vi "Main.vi"   [LabVIEW 2020]
doc: "Main interface to Dataflow DJ.\n\n<b>Execution System:</b> User Interface"
uses:
  Libraries/User Interface/Sub Panels Cluster.ctl
  Libraries/Track Info/Track Info FGV Enum.ctl
  Libraries/Audio Output/Audio Output Queue Type.ctl
  Libraries/Config File/Config Cluster.ctl
  Libraries/Track Info/Track Info.ctl
  <vilib>/Analysis/1siggen.llb/Ramp Pattern by Samples.vi
  Packed Libraries/Globals.lvlibp/Constants.vi
  <vilib>/Platform/TimedLoop/scheduler/LVUserAPI/_suppVIs/Create_SoftwareTrigger_TSource.vi
  Libraries/Audio Engine/Audio Engine.lvlib
  Libraries/Audio Output/Audio Output.lvlib
  Packed Libraries/Globals.lvlibp
  Libraries/User Interface/User Interface.lvlib
  Libraries/Config File/Config File.lvlib
  Libraries/Track Info/Track Info.lvlib
  <vilib>/Analysis/NI_AALBase.lvlib
  Plugin Interfaces/Controller Interface/Controller Interface.lvlibp/Controller Interface Class/Controller Interface.lvclass
  Libraries/Audio Recording/Audio Recording.lvlib
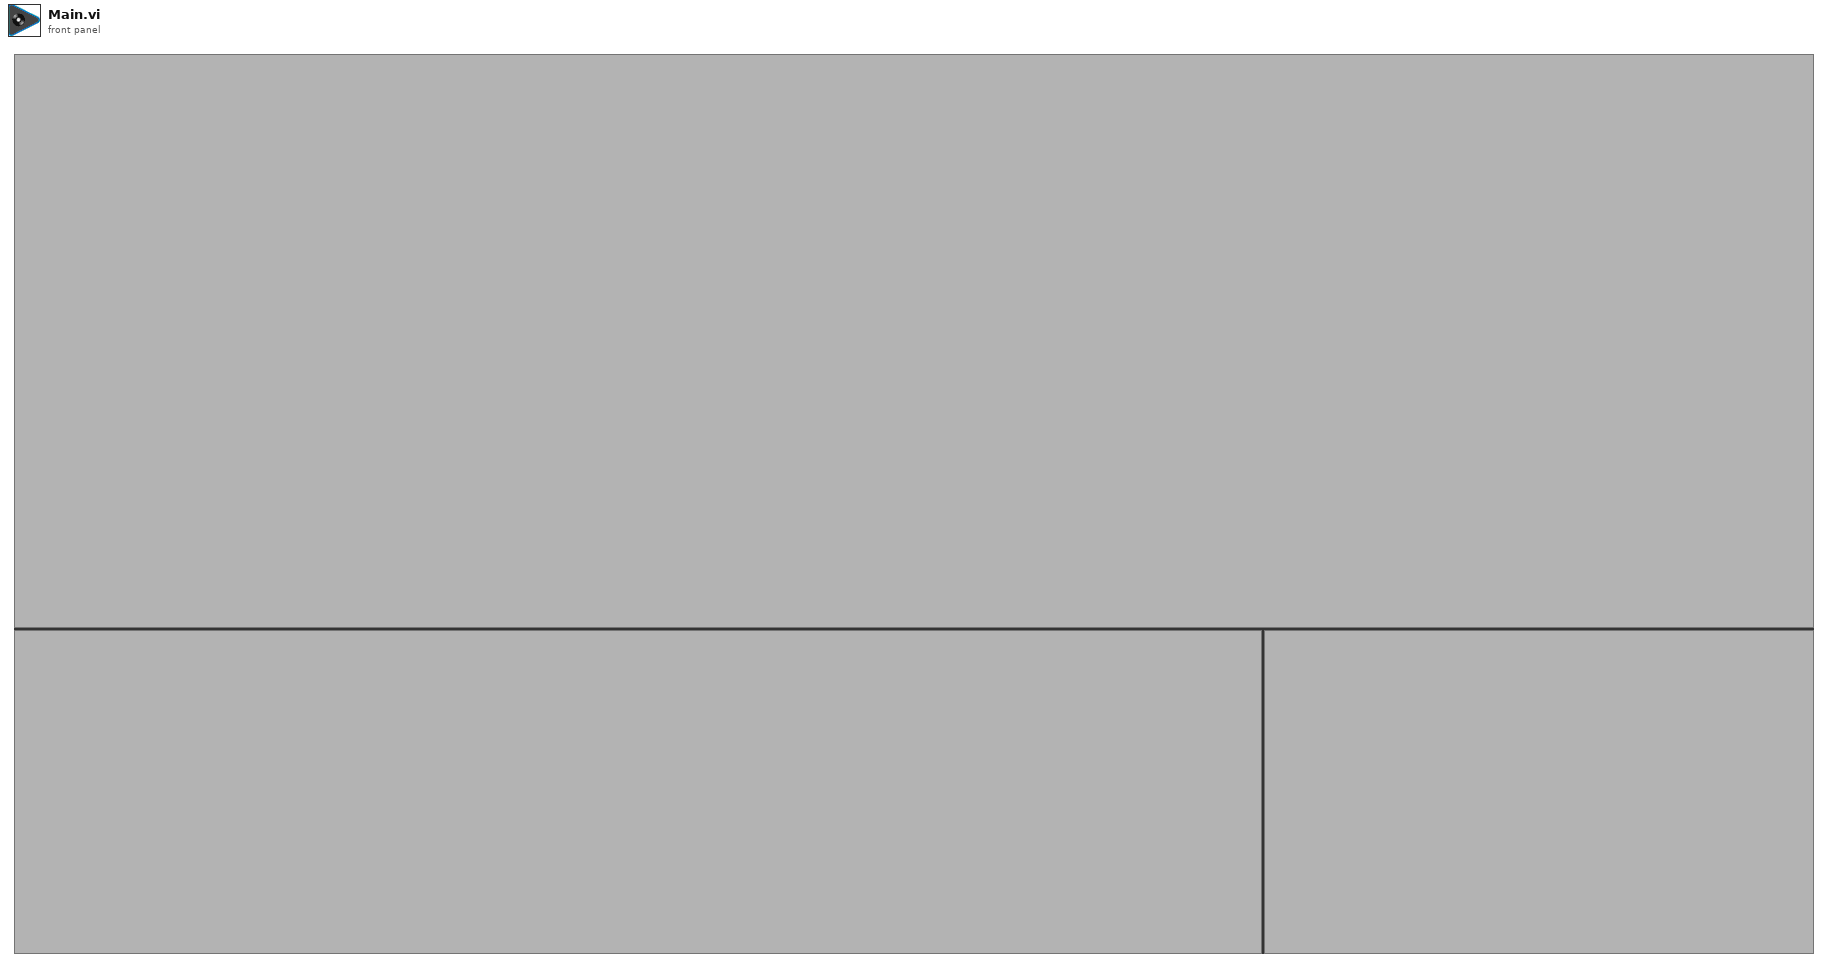
[diagram p1: front panel]
types:
  T1 = typedef "User Interface.lvlib/Sub Panels Cluster.ctl" = cluster{"DJ Interface":refnum<vi>, "File Browser":refnum<vi>, "Audio Config":refnum<vi>}
  T2 = typedef "Track Info.lvlib/Track Info FGV Enum.ctl" = enum16{"Init", "Update Track", "Update Multiple Tracks", "Get Track", "Get Multiple Tracks"}
  T3 = typedef "Config File.lvlib/Config Cluster.ctl" = cluster{"Track Info":T4[]}
  T4 = typedef "Track Info.lvlib/Track Info.ctl" = cluster{"Path":path, "Length (Samples)":i32, "Channels":i32, "Sample Rate (Hz)":i32, "BPM":dbl, "Cue Points (Samples)":i32[]}
  T5 = typedef "Audio Output.lvlib/Audio Output Queue Type.ctl" = cluster{"Master":waveform(i16)[], "Headphones":waveform(i16)[], "Start Time":dbl, "Record":bool}
  T6 = enum32{"invalid app kind", "Development System", "Run Time System", "Student Edition", "Embedded LabVIEW", "Evaluation", "Custom"}
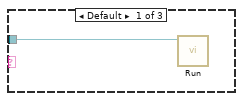
[diagram p2: hidden frame]
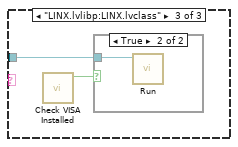
[diagram p4: hidden frame]
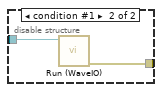
[diagram p7: hidden frame]
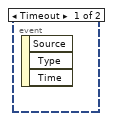
[diagram p8: hidden frame]
diagram:
  w12 = FALSE  # Shutdown
  # "#TODO\nOffload this checking logic to the class itself"
  # "Load WaveIO VIs programmatically\n\nif waveio.dll exists, then dynamically call VIs in waveio.llb\nif it doesn't exist, fall back to lvsound2.dll\n\nshould also address this issue"
  # "Startup order required\nAudio Processing\n- Setup message queues for all control messages from UI and hardware\n- Begin generating output data\nAutio Output\n- Setup message queue from audio config UI panel\nUser Interface (DJ Interface)\n- Setup message queue to receive UI changes\n- Scan all UI elements and send values and limits to Audio Processing\nHardware Controller\n- Setup hardware and read current IO state\n- Send IO state to Audio Processing, which will then relay changes back to UI\n\n#TODO Use named Notifiers to wait for each component to start up"
  # "EXECUTION SYSTEMS\n\nAudio Processing.Run.vi    Standard\nAudio Output.Run.vi    Instrument I/O\nMain.vi    User Interface\nUser Interface.DJ Interface.vi    User Interface\nUser Interface.File Browser.vi    User Interface\nUser Interface.Audio Config.vi    User Interface\nHardware Control.DAQmx Run.vi    Data Acquisition\nAudio File Input.Load Async.vi    Other 1"
  # "Dataflow DJ Mixer- A multichannel audio mixing application written entirely in LabVIEW, based on Dataflow DJ.\n    Copyright (C) 2020  Dataflow G\n    \n    This program is free software: you can redistribute it and/or modify\n    it under the terms of the GNU General Public License as published by\n    the Free Software Foundation, either version 3 of the License, or\n    (at your option) any later version.\n\n    This program is distributed in the hope that it will be useful,\n    but WITHOUT ANY WARRANTY; without even the implied warranty of\n    MERCHANTABILITY or FITNESS FOR A PARTICULAR PURPOSE.  See the\n    GNU General Public License for more details.\n\n    You should have received a copy of the GNU General Public License\n    along with this program.  If not, see <https://www.gnu.org/licenses/>.\n\nContact:\n    GitHub - https://github.com/dataflowg\n    Twitter - @Dataflow_G"
  # "If the WaveIO library is installed in external\\waveio_108, set WaveIO to TRUE in the Project's conditional disable symbols to use it here. \n\n#TODO\nAutomatically discover if WaveIO is available for development, maybe with a script or something."
  # "This is the main audio queue between the audio processing loop and audio output loop. It's a single element queue (SEQ) which contains the next block of audio data to be sent to both the master and headphone outputs. The block size is always Buffer Size (see global constant). Using a SEQ means the audio processing loop timing can be slaved to the audio output loop timing."
  # "Down, down, down. Would the fall NEVER come to an end!"
  n1 = flat-sequence {
    tunnel: [w35] -> w4
    tunnel: [w32] -> w3
    tunnel: [w28] -> _
    tunnel: [w28] -> w1
    frame #0 {
      # "Initialise Zero Buffer. This is sent to the soundcard when a track isn't loaded, is paused, or the headphone cue is disabled."
      n2 = global read "Constants.vi" "Buffer Size"() -> (w17:i32)
      n3 = global read "Constants.vi" "Channels"() -> (w18:i32)
      n4 = call "Track Info FGV.vi"("Track Info FGV Enum"=Track_Info_FGV_Enum."Init") -> ("error out"=w23:errorcluster)  [unwired: 7 in, 3 out]
      n5 = call-poly <vilib>:"Ramp Pattern.vi"("start"=0.0, "end"=1.0, "samples"=w17) -> ("Ramp Pattern"=w16:dbl[])  [unwired: 7 in, 1 out]
      n6 = call "Load Config.vi"("error in (no error)"=w23) -> ("Config"=w21:T3)  [unwired: 9 in, 1 out]
      n7 = Initialize Array(0.0, w18, w17) -> (w27:dbl[][])
      n8 = Unbundle By Name(w21) -> ("Track Info"=w25:T4[])
      n9 = Reverse 1D Array(array=w16) -> (reversed array=w15:dbl[])
      n10 = global write "Constants.vi" "Zero Buffer"(w27) -> ()
      n11 = global write "Constants.vi" "Ramp (Fade In)"(w16) -> ()
      n12 = global write "Constants.vi" "Ramp (Fade Out)"(w15) -> ()
      n13 = call "Track Info FGV.vi"("Track Info FGV Enum"=Track_Info_FGV_Enum."Update Multiple Tracks", "Multiple Track Info In"=w25) -> ()  [unwired: 6 in, 4 out]
    }
    frame #1 {
      w30 = T5 {"Master"=[], "Headphones"=[], "Start Time"=0.0, "Record"=FALSE}
      n14 = call-poly <vilib>:"Create Timing Source.vi"("trigger ID"=u8 0) -> ("timing source name"=w32:string)  [unwired: 9 in, 1 out]
      n15 = Obtain Queue(max queue size (-1, unlimited)=100, name (unnamed)="Recording", element data type=w30) -> (queue out=w28:refnum<queue>)  [unwired: 2 in, 2 out]
      n16 = Obtain Queue(max queue size (-1, unlimited)=1, name (unnamed)="Audio", element data type=w30) -> (queue out=w35:refnum<queue>)  [unwired: 2 in, 2 out]
    }
  }
  n17 = control-ref of="DJ Interface Sub Panel"() -> (w10:refnum<vi>)
  n18 = control-ref of="File Browser Sub Panel"() -> (w9:refnum<vi>)
  n19 = control-ref of="Audio Config Sub Panel"() -> (w8:refnum<vi>)
  n20 = Bundle By Name(cluster=T1 {"DJ Interface"=refnum, "File Browser"=refnum, "Audio Config"=refnum} ("Sub Panels"), "DJ Interface"=w10, "File Browser"=w9, "Audio Config"=w8) -> (w7:T1)
  n21 = control-ref of="This VI"() -> (w6:refnum<vi>)
  n22 = Create User Event(user event datatype=w12) -> (user event=w2:refnum<user-event>, error out=w5:errorcluster)  [unwired: 1 in]
  n23 = call "Insert Sub Panels.vi"("error in (no error)"=w5, "Shutdown Event"=w2, "Sub Panels"=w7, "Owning VI"=w6) -> ()  [unwired: 7 in, 1 out]
  n24 = disable-structure shown="Disabled" {
    disable-tunnel: w2 -> [w39 _]
    frame Disabled {
      n25 = call "Load Controller Plugins.vi"("Shutdown Event"=w39) -> ("Controller Plugins"=w38:refnum<class "Controller Interface.lvclass">[])  [unwired: 10 in]
      n26 = Array Size(array=w38) -> (size(s)=w37:i32)
      n27 = for {
        tunnel: w38 -> [w40] mode=indexing
        workers-P: w37 -> [_]
        n28 = call <vilib>:"Get LV Class Name.vi"("object"=w40) -> ("class name"=w41:string)  [unwired: 9 in, 1 out]
        n29 = case shown="\"DAQmx.lvlibp:DAQmx.lvclass\"" w41 {
          tunnel: w40 -> [w42 w44 w47]
          frame Default {
            n30 = call-dynamic "Run.vi"("Controller Interface in"=w42) -> ()  [unwired: 9 in, 2 out]
          }
          frame "DAQmx.lvlibp:DAQmx.lvclass" {
            n31 = call "Check DAQmx Installed.vi"() -> ("DAQmx Installed?"=w43:bool)  [unwired: 11 in]
            n32 = case shown="True" w43 {
              tunnel: w44 -> [_ w45]
              frame False {
              }
              frame True {
                n33 = call-dynamic "Run.vi"("Controller Interface in"=w45) -> ()  [unwired: 9 in, 2 out]
              }
            }
          }
          frame "LINX.lvlibp:LINX.lvclass" {
            n34 = call "Check VISA Installed.vi"() -> ("VISA Installed?"=w46:bool)  [unwired: 11 in]
            n35 = case shown="True" w46 {
              tunnel: w47 -> [_ w48]
              frame False {
              }
              frame True {
                n36 = call-dynamic "Run.vi"("Controller Interface in"=w48) -> ()  [unwired: 9 in, 2 out]
              }
            }
          }
        }
      }
    }
    frame Enabled {
    }
  }
  n37 = while {
    tunnel: w2 -> [w52]
    tunnel: w4 -> [w51]
    tunnel: w3 -> [w50]
    tunnel: w1 -> [w49]
    stop <- w53 stop-if-true
    n38 = event shown="[1] Panel Close?" {
      selector: _ -> [_ _]
      dyn-events: _ -> [_ _]
      timeout: _ -> [_ _]
      tunnel: [_ TRUE] -> w53
      tunnel: w52 -> [_ w70]
      tunnel: w51 -> [_ w64]
      tunnel: w50 -> [_ w58]
      tunnel: w49 -> [_ w54]
      event Timeout {
        n39 = event-data() -> ()  [unwired: 1 in, 3 out]
      }
      event Panel Close? {
        # "Write track info and config to disk on shutdown"
        # "Only close the panel if running under the run-time engine."
        n40 = event-data() -> ()  [unwired: 1 in, 4 out]
        n41 = Generate User Event(user event=w70, event data cluster=TRUE ("event data")) -> (user event out=w68:refnum<user-event>, error out=w67:errorcluster)  [unwired: 2 in]
        n42 = call "Track Info FGV.vi"("Track Info FGV Enum"=Track_Info_FGV_Enum."Get Multiple Tracks") -> ("Multiple Track Info Out"=w62:T4[])  [unwired: 7 in, 3 out]
        n43 = Destroy User Event(user event=w68, error in=w67) -> (error out=w63:errorcluster)
        n44 = Bundle By Name(cluster=T3 {"Track Info"=[]} ("Config"), "Track Info"=w62) -> (w61:T3)
        n45 = call "Save Config.vi"("Config"=w61) -> ()  [unwired: 10 in, 1 out]
        n46 = Release Queue(queue=w64, force destroy? (F)=TRUE, error in (no error)=w63) -> (error out=w56:errorcluster)  [unwired: 2 out]
        n47 = Release Queue(queue=w54, force destroy? (F)=TRUE, error in (no error)=w56) -> (error out=w55:errorcluster)  [unwired: 2 out]
        n48 = property class="App"() -> ("App.Kind"=w73:T6)  [unwired: 2 in, 2 out]
        n49 = call <vilib>:"Clear Timing Source.vi"("error in (no error)"=w55, "name"=w58) -> ()  [unwired: 8 in, 2 out]
        n50 = Not Equal?(x=w73, y=T6."Run Time System") -> (x != y?=w66:bool)
        n51 = event-data("Discard?"=w66) -> ()  [unwired: 1 in, 1 out]
      }
    }
  }
  n52 = disable-structure shown="Default" {
    disable-tunnel: w4 -> [w75 w77]
    disable-tunnel: [w74 w76] -> w14
    frame condition #0 (active) {
      n53 = call "Run (lvsound2).vi"("Audio Output Queue"=w75) -> ("error out"=w74:errorcluster)  [unwired: 10 in]
    }
    frame condition #1 {
      n54 = call "Run (WaveIO).vi"("Audio Output Queue"=w77) -> ("error out"=w76:errorcluster)  [unwired: 10 in]
    }
  }
  n55 = call "Run.vi"("Audio Data"=w1) -> ()  [unwired: 11 in]
  n56 = call "Run.vi"("Audio Record Queue"=w1, "Timing Source"=w3, "Audio Output Queue"=w4) -> ()  [unwired: 8 in, 1 out]
  n57 = call <vilib>:"General Error Handler.vi"("error in (no error)"=w14) -> ("error out"=w13:errorcluster)  [unwired: 10 in, 4 out]
  n58 = call ".vi"("error in (no escape)"=w13) -> ()
